vi "Close.vi"(8 "error in (no error)":errorcluster, 11 "Database Manager in":refnum<class "Database Manager.lvclass">) -> (0 "error out":errorcluster)   [LabVIEW 2019, in "HierDAL Library.lvlib" / "Database.lvlib" / "Database Manager.lvclass"]
uses:
  Database Manager.lvclass
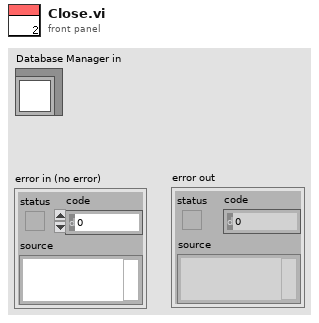
[diagram p1: front panel]
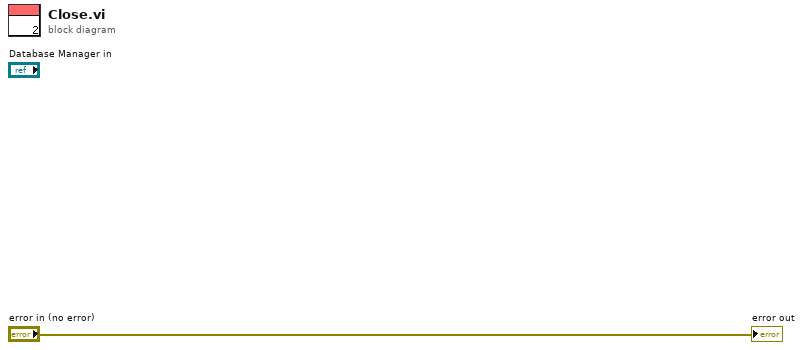
[diagram p0: block diagram]
diagram:
  "error out" <- "error in (no error)"
